vi "User Interface.vi"(8 "error in (no error)":errorcluster, 11 "User Interface in":refnum<class "User Interface.lvclass">) -> (0 "error out":errorcluster, 3 "User Interface out":refnum<class "User Interface.lvclass">)   [LabVIEW 2017, in "DSF Core.lvlib" / "Component Settings Editor.lvclass"]
uses:
  Component Settings Editor.lvclass
  User Interface.lvclass
  C:/Git/DSF/Core/Classes/User Interface/User Interface.lvclass
  User Interface.lvclass/User Interface.ctl
  User Interface Events/User Interface Events.lvclass/User Interface Events.ctl
  Component Settings Editor.lvclass/Component Settings Editor.ctl
  User Interface Handler/User Interface Handler.lvclass/User Interface Handler.ctl
  Get Events.vi
  User Interface Events/Generate Stop Event.vi
  User Interface Handler/User Interface Handler.lvclass
panel:
  in  "Components":i32(listbox)
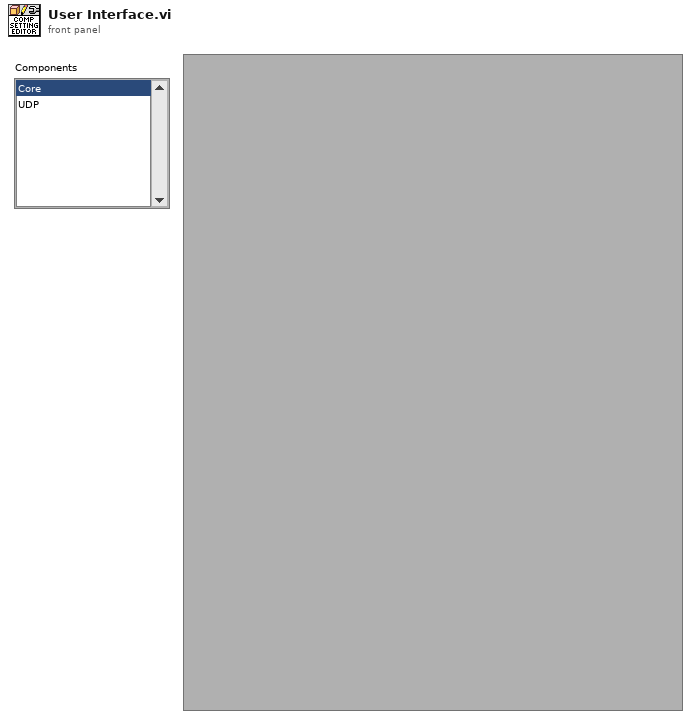
[diagram p1: front panel]
types:
  T1 = typedef "DSF Core.lvlib/User Interface Handler.lvclass/User Interface Ref.ctl" = refnum<vi>
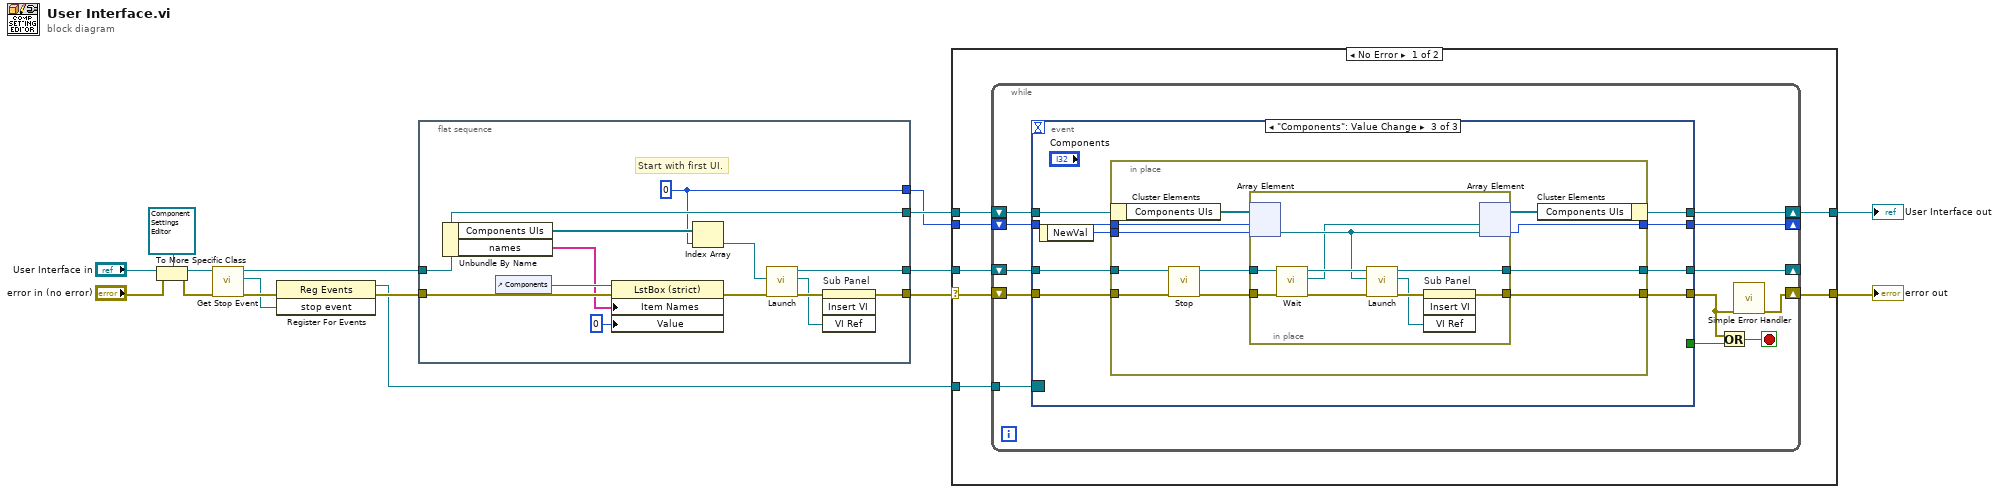
[diagram p0: block diagram]
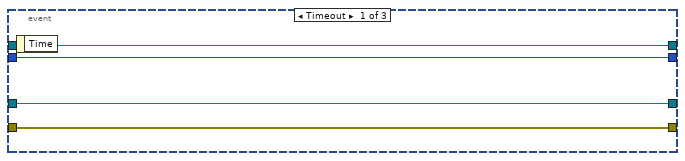
[diagram p2: hidden frame]
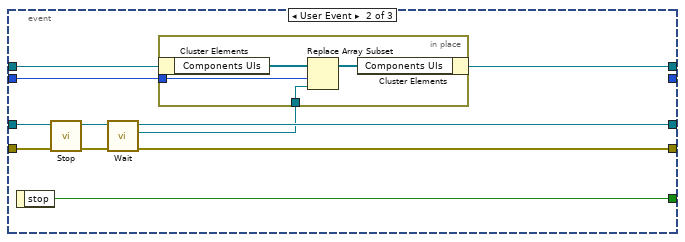
[diagram p3: hidden frame]
diagram:
  n1 = To More Specific Class(target class=refnum<class "Component Settings Editor.lvclass"> refnum ("DSF Core.lvlib:Plugin Settings Editor.lvclass"), reference="User Interface in", error in="error in (no error)") -> (specific class reference=w10:refnum<class "Component Settings Editor.lvclass">, error out=w9:errorcluster)
  n2 = call "Get Stop Event.vi"("error in (no error)"=w9, "User Interface in"=w10) -> ("error out"=w12:errorcluster, "stop event"=w11:refnum<user-event>, "User Interface out"=w4:refnum<class "Component Settings Editor.lvclass">)  [unwired: 7 in]
  n3 = register-events(error in=w12, w11) -> (reference out=w6:refnum<event-registration>, error out=w7:errorcluster)  [unwired: 1 in]
  n4 = flat-sequence {
    tunnel: w7 -> [w28]
    tunnel: [w25] -> w1
    tunnel: [w23] -> w5
    tunnel: w4 -> [w22]
    tunnel: [w22] -> w3
    tunnel: [w17] -> w2
    frame #0 {
      w17 = 0
      # "Start with first UI."
      n5 = Unbundle By Name(w22) -> ("Components UIs"=w21:refnum<class "User Interface.lvclass">[], "names"=w20:string[])
      n6 = control-ref of="Components"() -> (w29:refnum<vi>)
      n7 = property class="LstBox (strict)"(reference=w29, error in=w28, "Item Names"=w20, "Value"=0) -> (error out=w18:errorcluster)  [unwired: 1 out]
      n8 = Index Array(array=w21, index=w17) -> (element=w19:refnum<class "User Interface.lvclass">)
      n9 = call "Launch.vi"("error in (no error)"=w18, "User Interface"=w19) -> ("error out"=w26:errorcluster, "active vi"=w24:T1, "User Interface Handler out"=w23:refnum<class "User Interface Handler.lvclass">)  [unwired: 7 in]
      n10 = invoke on="Sub Panel" class="SubPnl" method="Insert VI"(error in=w26, "VI Ref"=w24) -> (error out=w25:errorcluster)  [unwired: 2 in, 3 out]
    }
  }
  n11 = case shown="No Error" w1 {
    selector: w1 -> [w30 w99]
    tunnel: [w36 w99] -> w16
    tunnel: [w35 w98] -> w13
    tunnel: w6 -> [w34 _]
    tunnel: w5 -> [w33 _]
    tunnel: w3 -> [w32 w98]
    tunnel: w2 -> [w31 _]
    frame No Error {
      n12 = while {
        tunnel: w34 -> [w48]
        shift-right: [w37] -> w36
        shift-left: w30 -> [w47]
        shift-right: [w43] -> _
        shift-left: w33 -> [w44]
        shift-right: [w41] -> w35
        shift-left: w32 -> [w42]
        shift-right: [w39] -> _
        shift-left: w31 -> [w40]
        stop <- w46 stop-if-true
        n13 = event shown="[2] \"Components\": Value Change" {
          selector: w48 -> [_ _ _]
          dyn-events: _ -> [_ _ _]
          timeout: _ -> [_ _ _]
          tunnel: [_ w63 _] -> w45
          tunnel: w47 -> [w52 w59 w71]
          tunnel: [w52 w58 w68] -> w38
          tunnel: w44 -> [w51 w60 w70]
          tunnel: [w51 w57 w69] -> w43
          tunnel: w42 -> [w50 w56 w76]
          tunnel: [w50 w53 w75] -> w41
          tunnel: w40 -> [w49 w55 w73]
          tunnel: [w49 _ w72] -> w39
          event Timeout {
            n14 = event-data() -> ()  [unwired: 1 in, 1 out]
          }
          event User Event {
            n15 = event-data() -> ("stop"=w63:bool)  [unwired: 1 in]
            n16 = call "Stop.vi"("error in (no error)"=w59, "User Interface Handler in"=w60) -> ("error out"=w61:errorcluster, "User Interface Handler out"=w62:refnum<class "User Interface Handler.lvclass">)  [unwired: 8 in]
            n17 = call "Wait.vi"("error in (no error)"=w61, "User Interface Handler in"=w62) -> ("error out"=w58:errorcluster, "User Interface"=w54:refnum<class "User Interface.lvclass">, "User Interface Handler out"=w57:refnum<class "User Interface Handler.lvclass">)  [unwired: 7 in]
            n18 = in-place {
              in-place-border: w55 -> [w65]
              in-place-border: w54 -> [w64]
              n19 = in-place-cluster #1(w56) -> ("Components UIs"=w67:refnum<class "User Interface.lvclass">[])
              n20 = Replace Array Subset(array=w67, new element=w64, index=w65) -> (w66:refnum<class "User Interface.lvclass">[])
              n21 = in-place-cluster #1("Components UIs"=w66) -> (w53:refnum<class "Component Settings Editor.lvclass">)
            }
          }
          event "Components": Value Change {
            n22 = event-data() -> ("NewVal"=w74:i32)  [unwired: 1 in]
            n23 = in-place {
              in-place-border: w73 -> [w87]
              in-place-border: w74 -> [w83]
              in-place-border: [w86] -> w72
              in-place-border: w71 -> [w79]
              in-place-border: w70 -> [w80]
              in-place-border: [w85] -> w69
              in-place-border: [w84] -> w68
              n24 = in-place-cluster #2(w76) -> ("Components UIs"=w82:refnum<class "User Interface.lvclass">[])
              n25 = call "Stop.vi"("error in (no error)"=w79, "User Interface Handler in"=w80) -> ("error out"=w78:errorcluster, "User Interface Handler out"=w77:refnum<class "User Interface Handler.lvclass">)  [unwired: 8 in]
              n26 = in-place {
                in-place-border: [w95] -> w85
                in-place-border: [w96] -> w84
                in-place-border: w78 -> [w89]
                in-place-border: w77 -> [w88]
                n27 = in-place-array #3(w82, w87, w83) -> (w91:refnum<class "User Interface.lvclass">)  [unwired: 1 out]
                n28 = call "Wait.vi"("error in (no error)"=w89, "User Interface Handler in"=w88) -> ("error out"=w93:errorcluster, "User Interface"=w90:refnum<class "User Interface.lvclass">, "User Interface Handler out"=w92:refnum<class "User Interface Handler.lvclass">)  [unwired: 7 in]
                n29 = call "Launch.vi"("error in (no error)"=w93, "User Interface"=w91, "User Interface Handler in"=w92) -> ("error out"=w97:errorcluster, "active vi"=w94:T1, "User Interface Handler out"=w95:refnum<class "User Interface Handler.lvclass">)  [unwired: 6 in]
                n30 = invoke on="Sub Panel" class="SubPnl" method="Insert VI"(error in=w97, "VI Ref"=w94) -> (error out=w96:errorcluster)  [unwired: 2 in, 3 out]
                n31 = in-place-array #3(w90, w91) -> (w81:refnum<class "User Interface.lvclass">[], w86:i32)  [unwired: 1 out]
              }
              n32 = in-place-cluster #2("Components UIs"=w81) -> (w75:refnum<class "Component Settings Editor.lvclass">)
            }
          }
        }
        n33 = Or(x=w38, y=w45) -> (x .or. y?=w46:bool)
        n34 = call <vilib>:"Simple Error Handler.vi"("error in (no error)"=w38) -> ("error out"=w37:errorcluster)  [unwired: 4 in, 4 out]
      }
    }
    frame Error {
    }
  }
  "error out" <- w16
  "User Interface out" <- w13
